vi "InitConnectionsArray.vi"(8 "error in (no error)":errorcluster, 11 "TCP_Server in":refnum<class "TCP_Server.lvclass">) -> (0 "error out":errorcluster, 3 "TCP_Server out":refnum<class "TCP_Server.lvclass">)   [LabVIEW 2023, in "TCP_Server.lvlib" / "TCP_Server.lvclass"]
uses:
  TCP_Server.lvclass
  TypeDeclarations/ServerConnection.ctl
  <vilib>/ActorFramework/Message Enqueuer/Message Enqueuer.lvclass
  TCP_Listener/TypeDefinitions/ConnectionInformation.ctl
  TCP_Server.lvclass/TCP_Server.ctl
  TCP_Server.lvlib
  TCP_Listener/TCP_Listener.lvlib
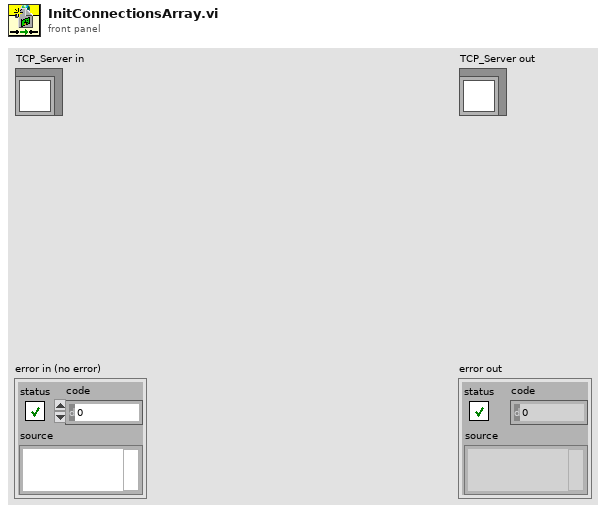
[diagram p1: front panel]
types:
  T1 = typedef "TCP_Server.lvlib/ServerConnection.ctl" = cluster{"Connection Handlers's Enqueuer":refnum<class "Message Enqueuer.lvclass">, "Connection Window's Enqueuer":refnum<class "Message Enqueuer.lvclass">, "Connection Information":T2}
  T2 = typedef "TCP_Listener.lvlib/ConnectionInformation.ctl" = cluster{"Connection number":i32, "Remote Address":string, "Remote Port":u16, "Connection ID":refnum<k5>}
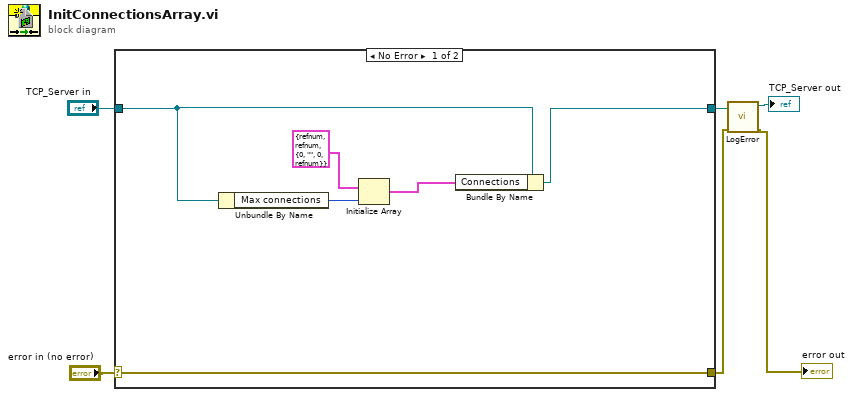
[diagram p0: block diagram]
diagram:
  n1 = case shown="No Error" "error in (no error)" {
    selector: "error in (no error)" -> [w12 w14]
    tunnel: [w12 w14] -> w2
    tunnel: [w7 w13] -> w4
    tunnel: "TCP_Server in" -> [w11 w13]
    frame No Error {
      n2 = Unbundle By Name(w11) -> ("Max connections"=w8:i32)
      n3 = Initialize Array(T1 {"Connection Handlers's Enqueuer"=refnum, "Connection Window's Enqueuer"=refnum, "Connection Information"={"Connection number"=0, "Remote Address"="", "Remote Port"=0, "Connection ID"=refnum}} ("Connection"), w8) -> (w9:T1[])
      n4 = Bundle By Name(cluster=w11, "Connections"=w9) -> (w7:refnum<class "TCP_Server.lvclass">)
    }
    frame Error {
    }
  }
  n5 = call "LogError.vi"("error in (no error)"=w2, "TCP_Server in"=w4) -> ("error out"=→"error out":errorcluster, "TCP_Server out"=→"TCP_Server out":refnum<class "TCP_Server.lvclass">)  [unwired: 8 in]
